vi "CALC_PAR_MOD_EXT.vi"(0 "VISA IN":refnum<visa-resource-name>, 1 "Measurement Parameter":string, 5 "error in":errorcluster, 7 "Channel":i32) -> (14 "VISA Out":refnum<visa-resource-name>, 19 "error out":errorcluster)   [LabVIEW 2018, in "PNA-X.lvlib"]
doc: "CALCulate<cnum>:PARameter:MODify:EXTended <param> \nNote: This command replaces CALC:PAR:MOD as it allows modification of measurements using \nexternal multiport testsets. \n(Write-only) Modifies a standard measurement using the same arguments as CALC:PAR:DEF:EXT. \nTo modify an FCA measurement, use CALC:CUST:MOD. \nSee Critical Note \nParameters \n<cnum> Channel number of the measurement. The selected measurement on that \nchannel will be changed. If unspecified, <cnum> is set to 1. \n<param> (String) New measurement parameter. Use the same <param> arguments as \nCALC:PAR:DEF:EXT. \nExamples SYST:PRESET \nCALC:PAR:DEF:EXT \"MyMeas\", \"S10_1\" \nCALC:PAR:SEL \"MyMeas\" \nCALC:PAR:MOD:EXT \"a4b4,1\" 'changes the selected S10_1 \nmeasurement to an a4/b4 measurement with source port 1 \nQuery Syntax Not Applicable \nDefault Not Applicable"
uses:
  PNA-X.lvlib
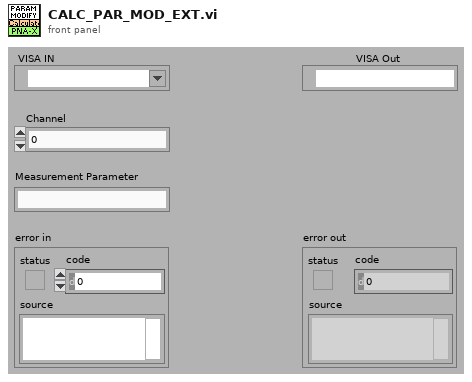
[diagram p1: front panel]
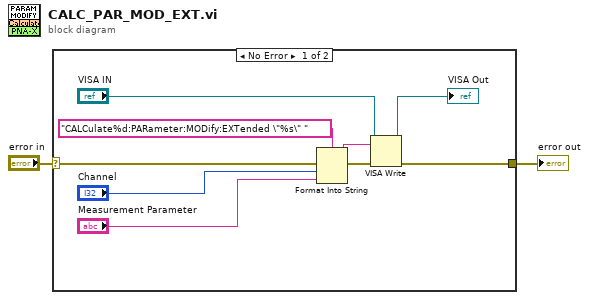
[diagram p0: block diagram]
diagram:
  n1 = case shown="No Error" "error in" {
    selector: "error in" -> [w11 w12]
    tunnel: [w6 w12] -> w1
    frame No Error {
      n2 = Format Into String(format string="CALCulate%d:PARameter:MODify:EXTended \"%s\" " ("Cmdline"), error in=w11, "Channel", "Measurement Parameter") -> (resulting string=w9:string, error out=w10:errorcluster)  [unwired: 1 in]
      n3 = VISA Write(VISA resource name="VISA IN", write buffer=w9, error in (no error)=w10) -> (VISA resource name out=→"VISA Out":refnum<visa-resource-name>, error out=w6:errorcluster)  [unwired: 1 out]
    }
    frame Error {
    }
  }
  "error out" <- w1
